vi "LV Server.vi"() -> ()   [LabVIEW 2018, in "Labview Python.lvlib"]
uses:
  Labview Python.lvlib
panel:
  out "# of Clients":i32
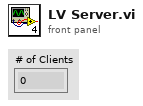
[diagram p1: front panel]
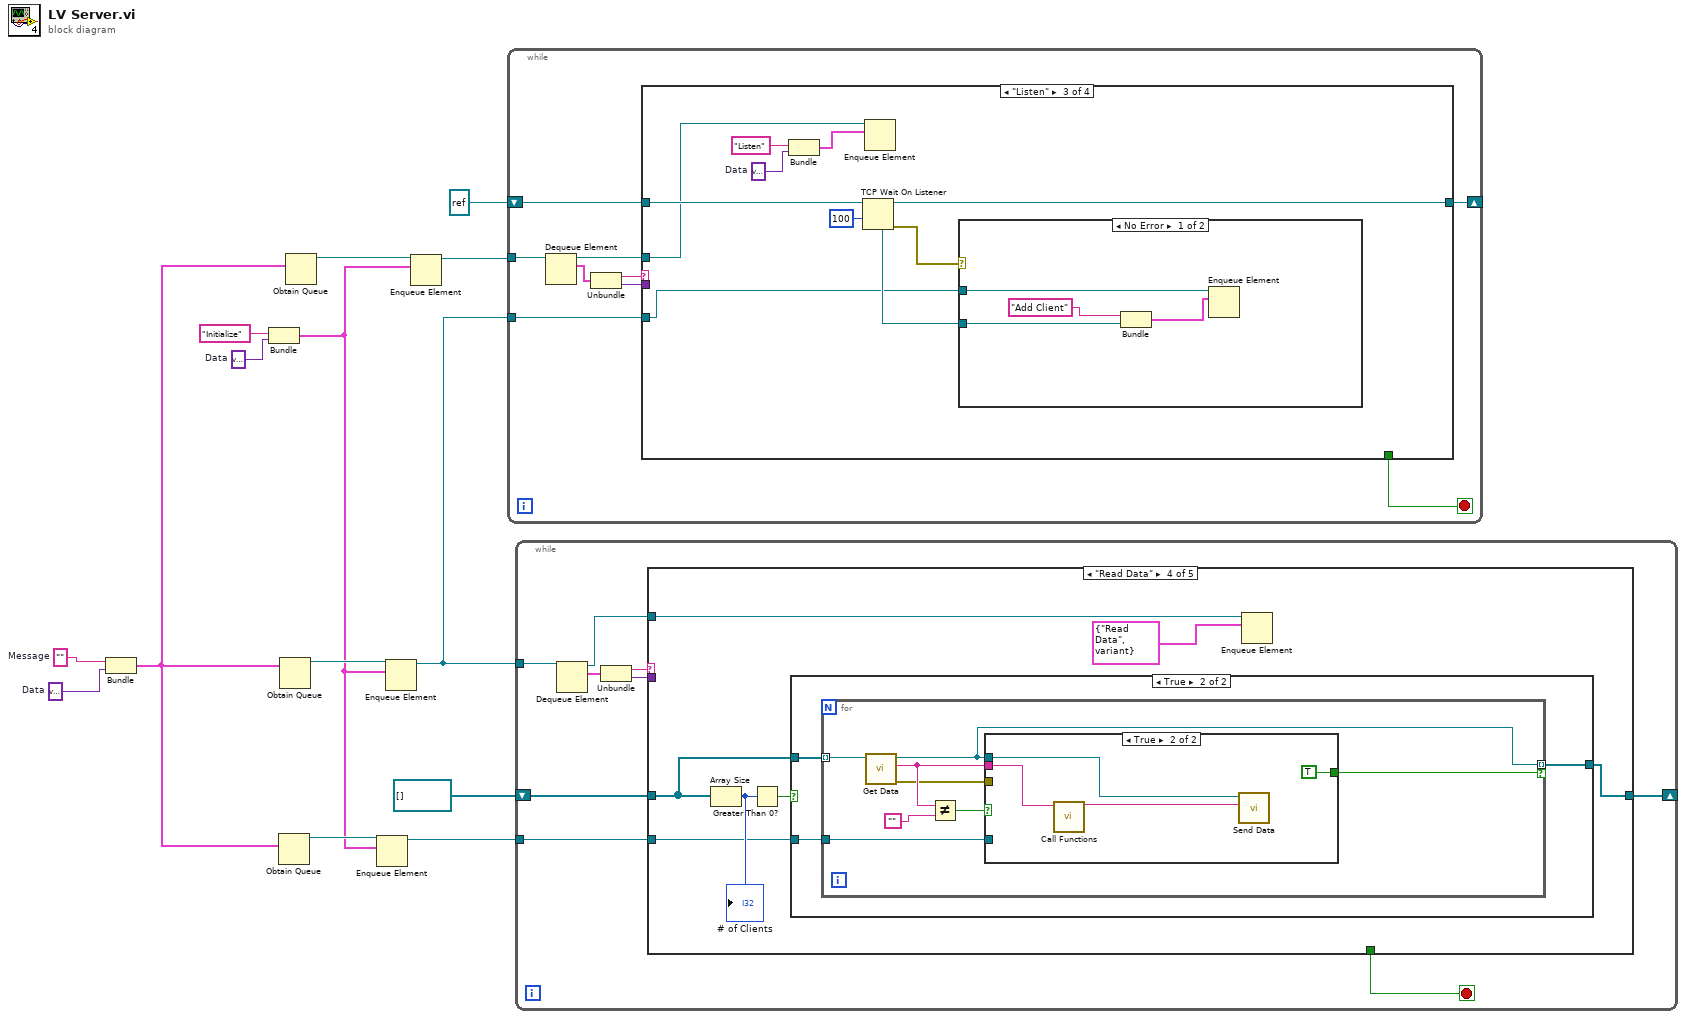
[diagram p0: block diagram]
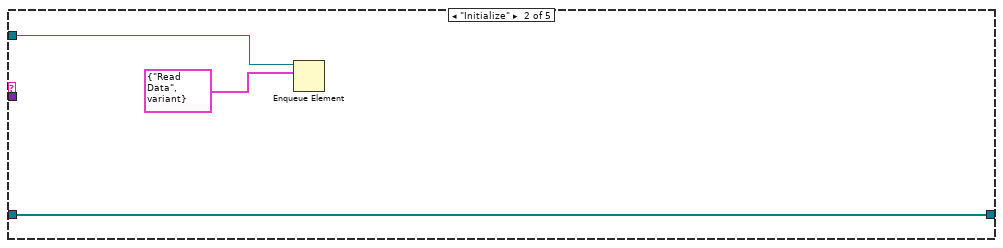
[diagram p3: hidden frame]
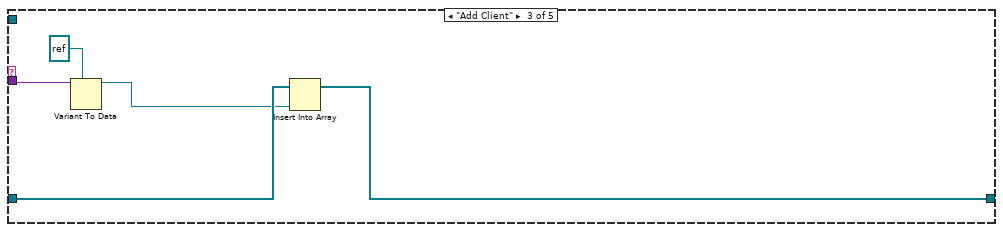
[diagram p4: hidden frame]
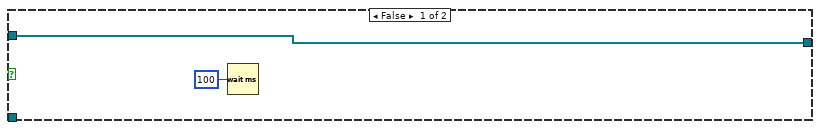
[diagram p5: hidden frame]
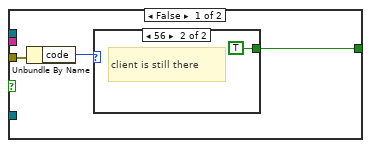
[diagram p6: hidden frame]
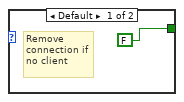
[diagram p7: hidden frame]
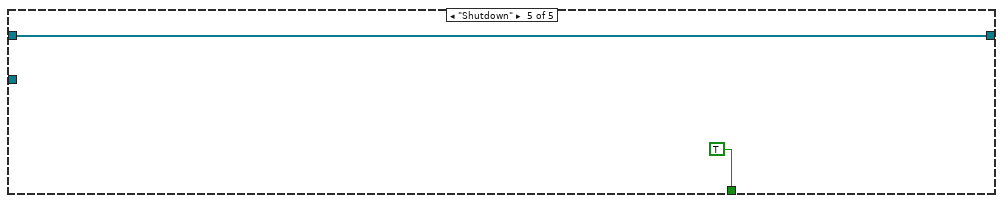
[diagram p8: hidden frame]
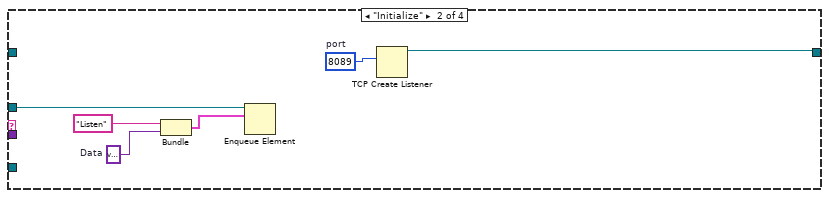
[diagram p10: hidden frame]
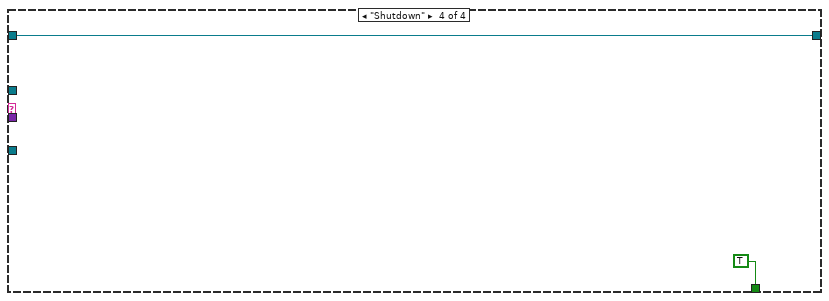
[diagram p12: hidden frame]
diagram:
  w6 = variant  # Data
  w8 = variant  # Data
  w9 = ""  # Message
  n1 = Bundle("Message"=w9, "Data"=w8) -> (w4:cluster{"Message":string, "Data":variant})  [unwired: 1 in]
  n2 = Bundle("element"="Initialize", "Data"=w6) -> (w2:cluster{"element":string, "Data":variant})  [unwired: 1 in]
  n3 = Obtain Queue(element data type=w4) -> (queue out=w3:refnum<queue>)  [unwired: 4 in, 2 out]
  n4 = Obtain Queue(element data type=w4) -> (queue out=w11:refnum<queue>)  [unwired: 4 in, 2 out]
  n5 = Obtain Queue(element data type=w4) -> (queue out=w14:refnum<queue>)  [unwired: 4 in, 2 out]
  n6 = Enqueue Element(queue=w3, element=w2) -> (queue out=w1:refnum<queue>)  [unwired: 2 in, 2 out]
  n7 = Enqueue Element(queue=w11, element=w2) -> (queue out=w5:refnum<queue>)  [unwired: 2 in, 2 out]
  n8 = Enqueue Element(queue=w14, element=w2) -> (queue out=w13:refnum<queue>)  [unwired: 2 in, 2 out]
  n9 = while {
    tunnel: w13 -> [w23]
    shift-right: [w20] -> _
    shift-left: refnum<k5> refnum ("listener ID in") -> [w21]
    tunnel: w5 -> [w16]
    stop <- w15 stop-if-true
    n10 = Dequeue Element(queue=w23) -> (queue out=w22:refnum<queue>, element=w19:cluster{"Message":string, "Data":variant})  [unwired: 2 in, 2 out]
    n11 = Unbundle(w19) -> ("Message"=w18:string, "Data"=w17:variant)
    n12 = case shown="\"Listen\"" w18 {
      tunnel: w22 -> [_ w30 w37 _]
      tunnel: w21 -> [w24 _ w40 w45]
      tunnel: [w24 w25 w39 w45] -> w20
      tunnel: w17 -> [_ _ _ _]
      tunnel: w16 -> [_ _ w31 _]
      tunnel: [_ _ _ TRUE] -> w15
      frame Default {
      }
      frame "Initialize" {
        w26 = u16 8089  # port
        w28 = variant  # Data
        n13 = Bundle("element"="Listen", "Data"=w28) -> (w27:cluster{"element":string, "Data":variant})  [unwired: 1 in]
        n14 = Enqueue Element(queue=w30, element=w27) -> ()  [unwired: 2 in, 3 out]
        n15 = TCP Create Listener(10:w26) -> (3:w25:refnum<k5>)  [unwired: 1 in, 5 out]
      }
      frame "Listen" {
        w35 = variant  # Data
        n16 = Bundle("element"="Listen", "Data"=w35) -> (w34:cluster{"element":string, "Data":variant})  [unwired: 1 in]
        n17 = TCP Wait On Listener(9:100 ("timeout ms (wait forever: -1)"), 11:w40) -> (0:w33:errorcluster, 3:w39:refnum<k5>, 4:w32:refnum<k5>)  [unwired: 1 in, 3 out]
        n18 = Enqueue Element(queue=w37, element=w34) -> ()  [unwired: 2 in, 3 out]
        n19 = case shown="No Error" w33 {
          tunnel: w32 -> [w42 _]
          tunnel: w31 -> [w41 _]
          frame No Error {
            n20 = Bundle("Add Client", "listener ID in"=w42) -> (w44:cluster{string, "listener ID in":refnum<k5>})  [unwired: 1 in]
            n21 = Enqueue Element(queue=w41, element=w44) -> ()  [unwired: 2 in, 3 out]
          }
          frame Error {
          }
        }
      }
      frame "Shutdown" {
      }
    }
  }
  n22 = while {
    tunnel: w5 -> [w55]
    shift-right: [w50] -> _
    shift-left: refnum<k5>[] [] ("connection IDs In") -> [w51]
    tunnel: w1 -> [w48]
    stop <- w47 stop-if-true
    n23 = Dequeue Element(queue=w55) -> (queue out=w49:refnum<queue>, element=w54:cluster{"Message":string, "Data":variant})  [unwired: 2 in, 2 out]
    n24 = Unbundle(w54) -> ("Message"=w53:string, "Data"=w52:variant)
    n25 = case shown="\"Read Data\"" w53 {
      tunnel: w52 -> [_ _ w64 _ _]
      tunnel: w51 -> [w56 w59 w62 w67 w95]
      tunnel: [w56 w59 w60 w65 w95] -> w50
      tunnel: w49 -> [_ w57 _ w69 _]
      tunnel: w48 -> [_ _ _ w66 _]
      tunnel: [_ _ _ _ TRUE] -> w47
      frame Default {
      }
      frame "Initialize" {
        n26 = Enqueue Element(queue=w57, element=cluster{"Message":string, "Data":variant} {"Message"="Read Data", "Data"=variant}) -> ()  [unwired: 2 in, 3 out]
      }
      frame "Add Client" {
        n27 = Variant To Data(type=refnum<k5> refnum ("listener ID in"), Variant=w64) -> (data=w61:refnum<k5>)  [unwired: 1 in, 1 out]
        n28 = Insert Into Array(array=w62, new element=w61) -> (w60:refnum<k5>[])  [unwired: 1 in]
      }
      frame "Read Data" {
        n29 = Array Size(array=w67) -> (size(s)=w71:i32)
        "# of Clients" <- w71
        n30 = Greater Than 0?(x=w71) -> (x > 0?=w70:bool)
        n31 = case shown="True" w70 {
          tunnel: w67 -> [w72 w76]
          tunnel: [w72 w75] -> w65
          tunnel: w66 -> [_ w74]
          frame False {
            n32 = Wait (ms)(milliseconds to wait=u32 100) -> ()  [unwired: 1 out]
          }
          frame True {
            n33 = for {
              tunnel: w76 -> [w81] mode=indexing
              tunnel: [w84] -> w75 mode=indexing if=w83
              tunnel: w74 -> [w82]
              n34 = call "Get Data.vi"("connection ID In"=w81) -> ("error out"=w77:errorcluster, "Data"=w80:string, "connection ID Out"=w84:refnum<k5>)  [unwired: 8 in]
              n35 = Not Equal?(x=w80, y="") -> (x != y?=w78:bool)
              n36 = case shown="True" w78 {
                tunnel: w80 -> [_ w92]
                tunnel: w84 -> [_ w91]
                tunnel: [w85 TRUE] -> w83
                tunnel: w82 -> [_ _]
                tunnel: w77 -> [w87 _]
                frame False {
                  n37 = Unbundle By Name(w87) -> ("code"=w86:i32)
                  n38 = case shown="56" w86 {
                    tunnel: [FALSE TRUE] -> w85
                    frame Default {
                      # "Remove connection if no client"
                    }
                    frame 56 {
                      # "client is still there"
                    }
                  }
                }
                frame True {
                  n39 = call "Call Functions.vi"("Data In"=w92) -> ("Data Out"=w90:string)  [unwired: 10 in]
                  n40 = call "Send Data.vi"("Data"=w90, "connection ID In"=w91) -> ()  [unwired: 8 in, 2 out]
                }
              }
            }
          }
        }
        n41 = Enqueue Element(queue=w69, element=cluster{"Message":string, "Data":variant} {"Message"="Read Data", "Data"=variant}) -> ()  [unwired: 2 in, 3 out]
      }
      frame "Shutdown" {
      }
    }
  }
